vi "vi1.vi"() -> ()   [LabVIEW 2018]
panel:
  in  "stop":bool
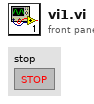
[diagram p1: front panel]
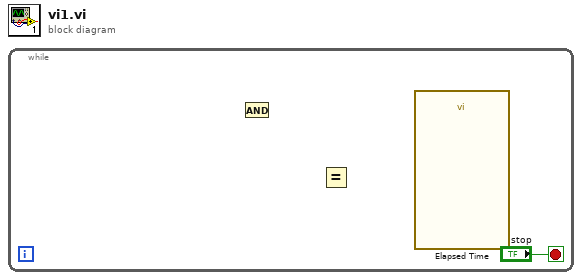
[diagram p0: block diagram]
diagram:
  n1 = while {
    stop <- "stop" stop-if-true
    n2 = And() -> ()  [unwired: 2 in, 1 out]
    n3 = Equal?() -> ()  [unwired: 2 in, 1 out]
    n4 = call "Elapsed Time"() -> ()  [unwired: 12 in, 8 out]
  }
